vi "Test CAN IO Class.vi"(7 "Type(5=DBL)":u8=255, 8 "error in (no error)":errorcluster, 10 "TLV Path(Tesla provided path)":path=path "C:/code/projects/Tesla/Tesla_testla/Ben submission/Data Files/test3.bin") -> (0 "error out":errorcluster, 2 "Passed?":bool)   [LabVIEW 2013]
uses:
  CAN IO_class/CAN IO.lvclass
panel:
  out "Numeric":i32
  out "Array":dbl[](array[numeric])
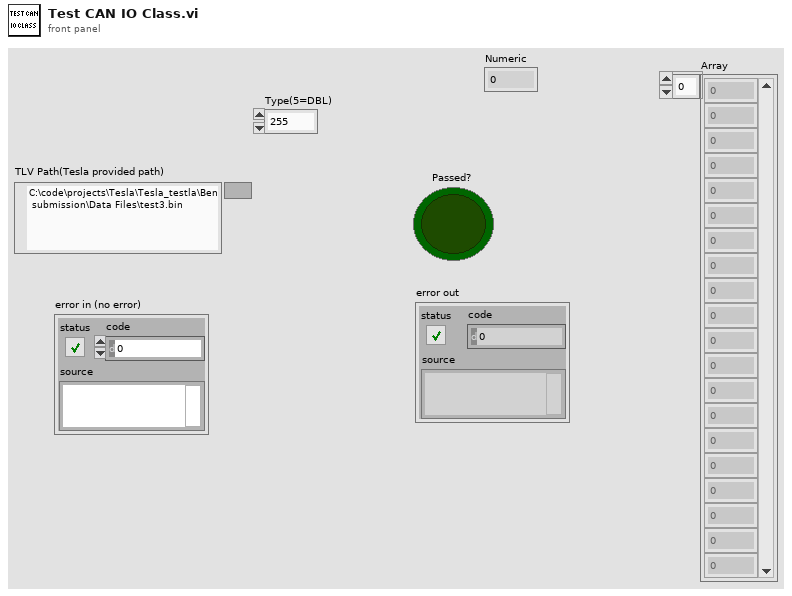
[diagram p1: front panel]
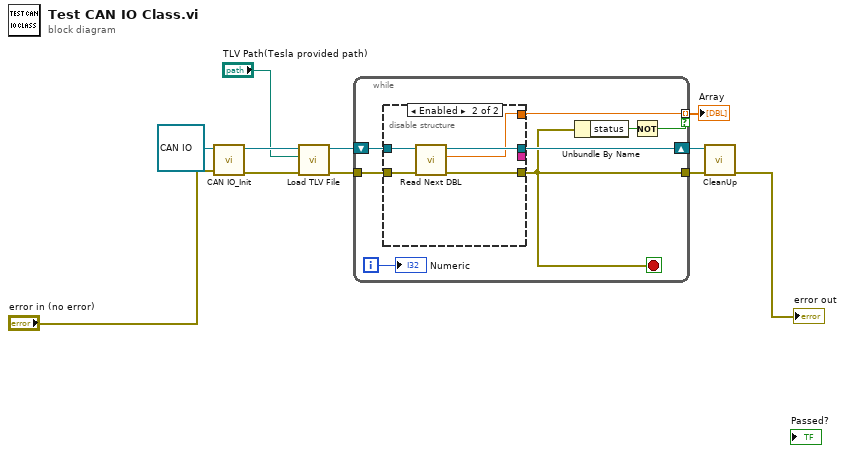
[diagram p0: block diagram]
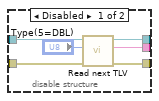
[diagram p2: hidden frame]
diagram:
  n1 = call "CAN IO_Init.vi"("error in (no error)"="error in (no error)", "object in"=refnum<class "CAN IO.lvclass"> refnum) -> ("error out"=w10:errorcluster, "object out"=w11:refnum<class "CAN IO.lvclass">)  [unwired: 8 in]
  n2 = call "Load TLV File.vi"("error in (no error)"=w10, "TLV Path"="TLV Path(Tesla provided path)", "object in"=w11) -> ("error out"=w8:errorcluster, "object out"=w9:refnum<class "CAN IO.lvclass">)  [unwired: 7 in]
  n3 = while {
    tunnel: w8 -> [w18]
    tunnel: [w15] -> w4
    shift-right: [w17] -> w5
    shift-left: w9 -> [w19]
    tunnel: [w16] -> w1 mode=indexing if=w13
    i -> [w12]
    stop <- w15 stop-if-true
    n4 = disable-structure shown="Enabled" {
      disable-tunnel: w19 -> [w25 w30]
      disable-tunnel: w18 -> [w24 w29]
      disable-tunnel: [w23 w28] -> w17
      disable-tunnel: [w22 w26] -> w15
      disable-tunnel: [w21 _] -> _
      disable-tunnel: [_ w27] -> w16
      frame Disabled {
        n5 = call-dynamic "Read next TLV.vi"("error in (no error)"=w24, "Type(255=next available)"="Type(5=DBL)", "object in"=w25) -> ("error out"=w22:errorcluster, "TLV Payload"=w21:string, "object out"=w23:refnum<class "CAN IO.lvclass">)  [unwired: 6 in]
      }
      frame Enabled {
        n6 = call "Read Next DBL.vi"("error in (no error)"=w29, "object in"=w30) -> ("error out"=w26:errorcluster, "Value Read"=w27:dbl, "object out"=w28:refnum<class "CAN IO.lvclass">)  [unwired: 7 in]
      }
    }
    n7 = Unbundle By Name(w15) -> ("status"=w14:bool)
    n8 = Not(x=w14) -> (.not. x?=w13:bool)
    "Numeric" <- w12
  }
  "Array" <- w1
  n9 = call-dynamic "CleanUp.vi"("error in (no error)"=w4, "object in"=w5) -> ("error out"=→"error out":errorcluster)  [unwired: 8 in, 1 out]
